vi "mes参数配置.vi"() -> (2 "确定":bool)   [LabVIEW 2020]
uses:
  Global.vi
panel:
  in  "取消":bool
  in  "确定":bool
  in  "MES参数":T1
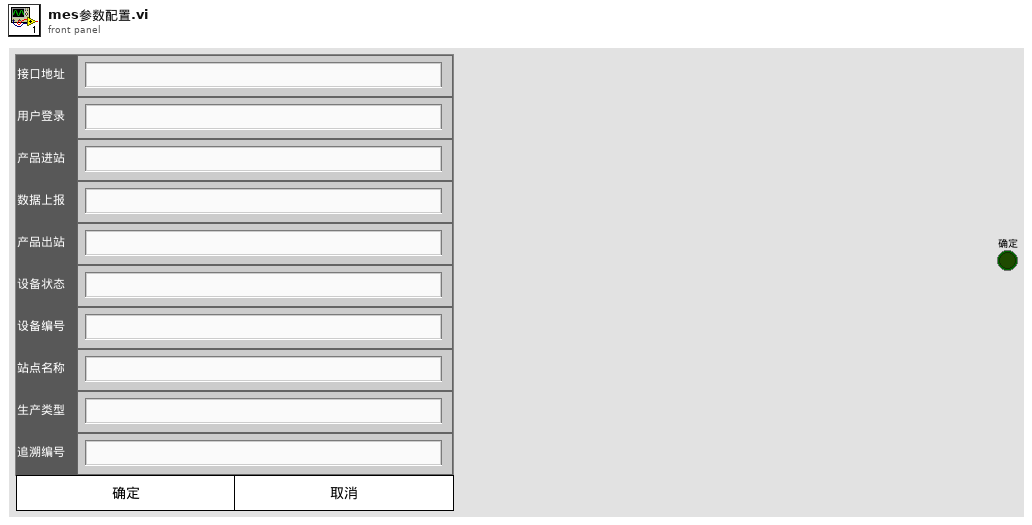
[diagram p1: front panel]
types:
  T1 = cluster{"接口地址":string, "用户登录":string, "产品进站":string, "数据上报":string, "产品出站":string, "设备状态":string, "设备编号":string, "站点名称":string, "生产类型":string, "追溯编号":string}
  T2 = cluster{"接口地址(URL)":string, "用户登录":string, "产品进站":string, "参数采集":string, "产品出站":string, "设备状态":string, "设备编号(equipNum)":string, "站点名称(siteCode)":string, "生产类型(productType)":string, "追溯编号(traceCode)":string}
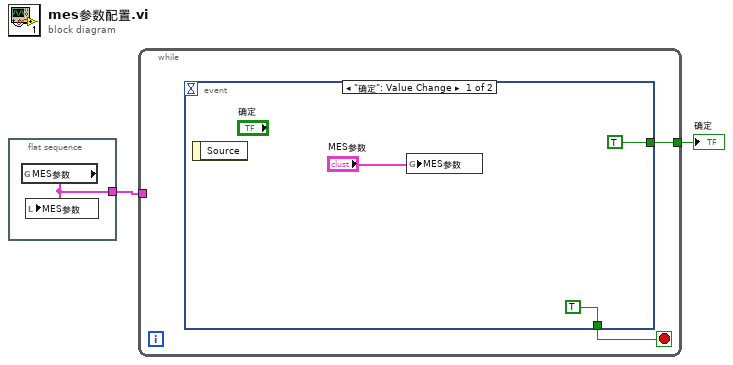
[diagram p0: block diagram]
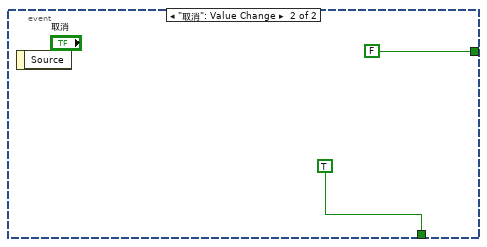
[diagram p2: hidden frame]
diagram:
  n1 = flat-sequence {
    tunnel: [w3] -> w2
    frame #0 {
      n2 = global read "Global.vi" "MES参数"() -> (w3:T2)
      n3 = local write "MES参数"(w3) -> ()
    }
  }
  n4 = while {
    tunnel: w2 -> [_]
    tunnel: [w4] -> w1
    stop <- w5 stop-if-true
    n5 = event shown="[0] \"确定\": Value Change" {
      selector: _ -> [_ _]
      dyn-events: _ -> [_ _]
      timeout: _ -> [_ _]
      tunnel: [TRUE TRUE] -> w5
      tunnel: [TRUE FALSE] -> w4
      event "确定": Value Change {
        n6 = event-data() -> ()  [unwired: 1 in, 1 out]
        n7 = global write "Global.vi" "MES参数"("MES参数") -> ()
      }
      event "取消": Value Change {
        n8 = event-data() -> ()  [unwired: 1 in, 1 out]
      }
    }
  }
  "确定" <- w1
